vi "Calculate dBdt.vi"(11 "B Field (T)":dbl) -> (3 "dB/dt (T/min)":dbl)   [LabVIEW 2019, in "Transport.lvclass"]
uses:
  Transport.lvclass
  <vilib>/ptbypt/NI_PtbyPt.lvlib
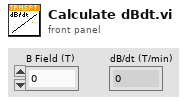
[diagram p1: front panel]
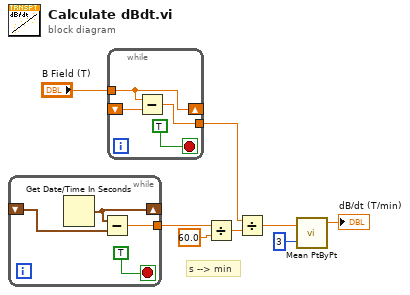
[diagram p0: block diagram]
diagram:
  # "s --> min"
  n1 = while {
    shift-right: [w10] -> _
    shift-left: _ -> [w9]
    tunnel: [w11] -> w2
    stop <- TRUE stop-if-true
    n2 = Get Date/Time In Seconds() -> (seconds since 1Jan1904=w10:timestamp)
    n3 = Subtract(x=w10, y=w9) -> (x-y=w11:dbl)
  }
  n4 = while {
    shift-right: [w13] -> _
    shift-left: _ -> [w14]
    tunnel: [w15] -> w5
    tunnel: "B Field (T)" -> [w13]
    stop <- TRUE stop-if-true
    n5 = Subtract(x=w13, y=w14) -> (x-y=w15:dbl)
  }
  n6 = Divide(x=w2, y=60.0) -> (x/y=w1:dbl)
  n7 = Divide(x=w5, y=w1) -> (x/y=w6:dbl)
  n8 = call <vilib>:"Mean PtByPt.vi"("x"=w6, "sample length"=3) -> ("mean"=→"dB/dt (T/min)":dbl)  [unwired: 2 in, 1 out]
